vi "SetParam.vi"(8 "error in (no error)":errorcluster caption="entrée d'erreur (pas d'erreur)", 10 "make_regression":T1={"n_samples"=100, "n_features"=100, "n_informative"=10, "n_targets"=1, "bias"=0.0, "effective_rank"="None", "tail_strength"=0.5, "noise"=0.0, "shuffle"=TRUE, "random_state"=-1, "Returns"="X"} {"tail_strength" min=0.0 max=1.0; "n_targets" min=1; "n_features" min=1; "n_samples" min=1}, 11 "Regression.lvclass":refnum<class "Regression.lvclass">) -> (0 "error out":errorcluster caption="sortie d'erreur", 3 "Regression.lvclass":refnum<class "Regression.lvclass">)   [LabVIEW 2020, in "Regression.lvclass"]
doc: "Set Parameters"
uses:
  Regression.lvclass
  Regression.lvclass/Regression.ctl
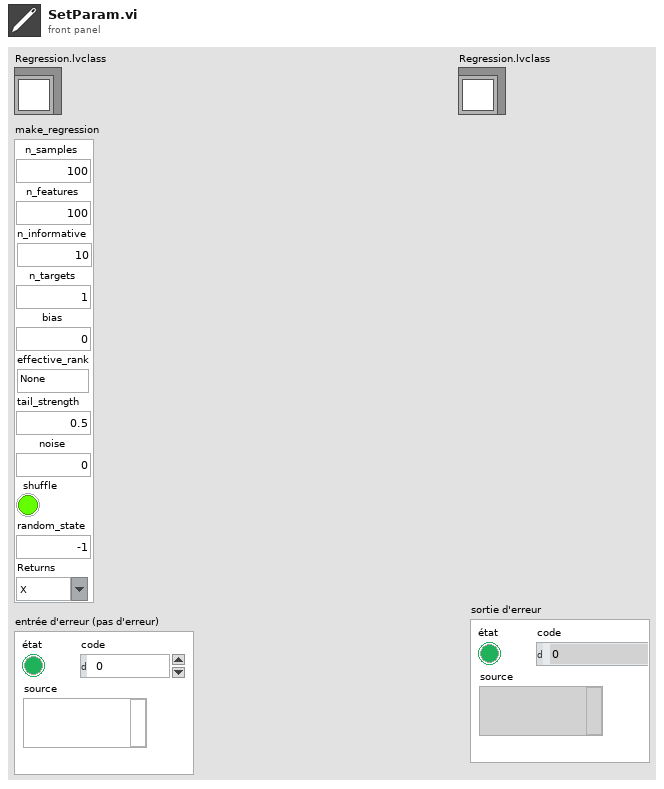
[diagram p1: front panel]
types:
  T1 = cluster{"n_samples":u32, "n_features":u32, "n_informative":u32, "n_targets":u32, "bias":dbl, "effective_rank":string, "tail_strength":dbl, "noise":dbl, "shuffle":bool, "random_state":i32, "Returns":string}
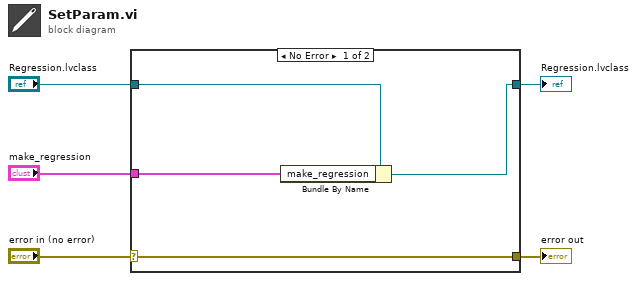
[diagram p0: block diagram]
diagram:
  n1 = case shown="No Error" "error in (no error)" {
    selector: "error in (no error)" -> [w9 w10]
    tunnel: [w9 w10] -> w4
    tunnel: [w7 w11] -> w2
    tunnel: "Regression.lvclass" -> [w8 w11]
    tunnel: "make_regression" -> [w6 _]
    frame No Error {
      n2 = Bundle By Name(cluster=w8, "make_regression"=w6) -> (w7:refnum<class "Regression.lvclass">)
    }
    frame Error {
    }
  }
  "error out" <- w4
  "Regression.lvclass" <- w2
